vi "DHE_GetnightID.vi"(8 "error in (no error)":errorcluster) -> (0 "error out":errorcluster, 2 "nightID":string)   [LabVIEW 2016]
uses:
  DBSHAND/private/vis/DatabaseHand_Element_Get(bool).vi
  DBSHAND/private/vis/DatabaseHand_Element_Get(string).vi
  DBSHAND/private/vis/DatabaseHand_Element_Set(string).vi
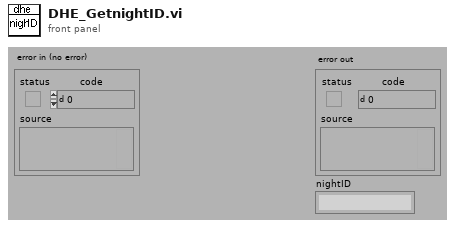
[diagram p1: front panel]
types:
  T1 = typedef "DatabaseHand_RefNum.ctl" = refnum<vi>
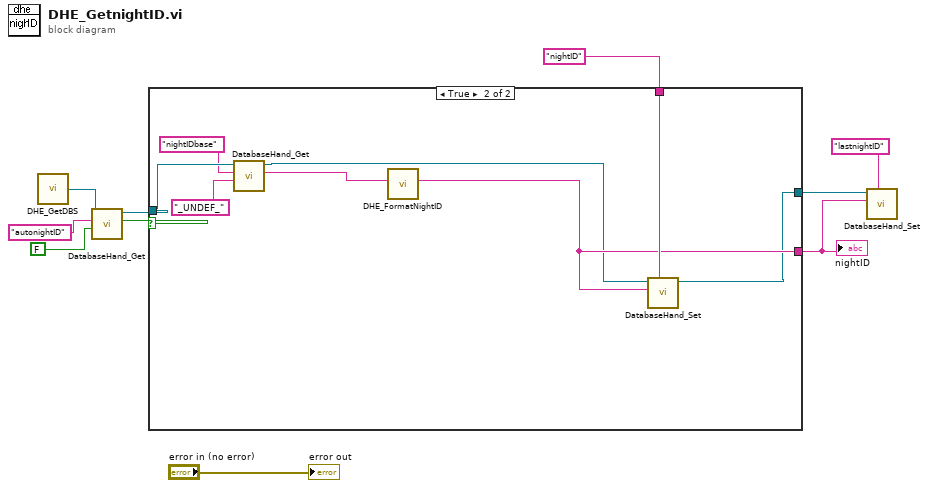
[diagram p0: block diagram]
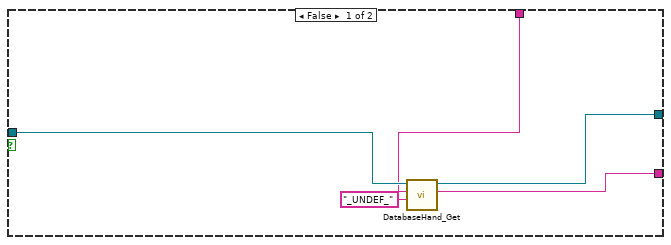
[diagram p2: hidden frame]
diagram:
  n1 = call "DHE_GetDBS.vi"() -> ("DHE_DBSRef"=w10:T1)  [unwired: 9 out]
  n2 = call-poly "DatabaseHand_Get.vi"("default value"=FALSE, "name"="autonightID", "Database RefNum in"=w10) -> ("value"=w7:bool, "Database RefNum out"=w6:T1)  [unwired: 2 in, 5 out]
  n3 = case shown="True" w7 {
    tunnel: w6 -> [w15 w23]
    tunnel: [w13 w18] -> w2
    tunnel: "nightID" ("name") -> [w14 w20]
    tunnel: [w12 w17] -> w1
    frame False {
      n4 = call-poly "DatabaseHand_Get.vi"("default value"="_UNDEF_", "name"=w14, "Database RefNum in"=w15) -> ("value"=w13:string, "Database RefNum out"=w12:T1)  [unwired: 2 in, 5 out]
    }
    frame True {
      n5 = call-poly "DatabaseHand_Get.vi"("default value"="_UNDEF_", "name"="nightIDbase", "Database RefNum in"=w23) -> ("value"=w19:string, "Database RefNum out"=w16:T1)  [unwired: 2 in, 5 out]
      n6 = call "DHE_FormatNightID.vi"("IDbase in"=w19) -> ("expID out"=w18:string)  [unwired: 1 in, 9 out]
      n7 = call-poly "DatabaseHand_Set.vi"("name"=w20, "value"=w18, "Database RefNum in"=w16) -> ("Database RefNum out"=w17:T1)  [unwired: 5 in, 3 out]
    }
  }
  "nightID" <- w2
  n8 = call-poly "DatabaseHand_Set.vi"("name"="lastnightID", "value"=w2, "Database RefNum in"=w1) -> ()  [unwired: 5 in, 4 out]
  "error out" <- "error in (no error)"
